vi "Launch Service Mode.vi"(8 "error in (no error)":errorcluster, 11 "Top in":refnum<class "Top.lvclass">) -> (0 "error out":errorcluster, 3 "Top out":refnum<class "Top.lvclass">)   [LabVIEW 2021, in "Top.lvlib" / "Top.lvclass"]
uses:
  Top.lvclass
  Top.lvclass/Top.ctl
  <vilib>/MGI/Panel Manager/Panel Actor/Panel Actor/Panel Actor.lvclass
  <vilib>/MGI/Panel Manager/Panel/Panel.lvlib
  <vilib>/MGI/Panel Manager/Panel/Panel/Window/Window.vi
  <vilib>/MGI/Panel Manager/Panel/Panel/Window/Window.lvclass
  Service/Service.lvclass
  C:/Program Files/National Instruments/LabVIEW 2021/vi.lib/MGI/Panel Manager/Panel/Panel/Panel.lvclass
  C:/Program Files/National Instruments/LabVIEW 2021/vi.lib/MGI/Panel Manager/Panel/Panel/Window/Window.lvclass
  C:/Program Files/National Instruments/LabVIEW 2021/vi.lib/MGI/Panel Manager/Panel Actor/Panel Actor/Panel Actor.lvclass
  C:/Program Files/National Instruments/LabVIEW 2021/vi.lib/ActorFramework/Actor/Actor.lvclass
  C:/git/IV-Curve-PH316/Source/Service/Service.lvclass
  C:/git/IV-Curve-PH316/Source/Top/Top.lvclass
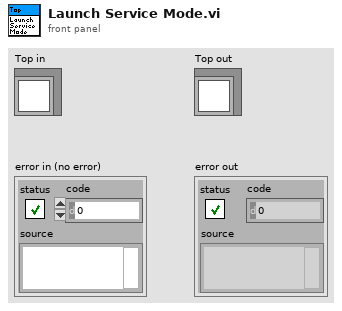
[diagram p1: front panel]
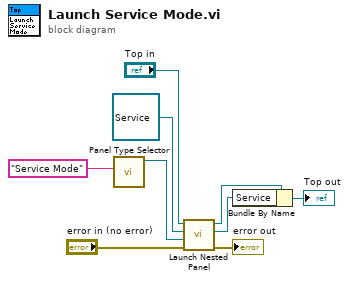
[diagram p0: block diagram]
diagram:
  n1 = call-poly <vilib>:"Panel Type Selector.vi"("Default Title"="Service Mode") -> ("Window out"=w8:refnum<class "Window.lvclass">)  [unwired: 9 in, 1 out]
  n2 = call <vilib>:"Launch Nested Panel.vi"("error in (no error)"="error in (no error)", "Panel"=w8, "Nested Panel Actor"=refnum<class "Service.lvclass"> refnum ("Service.lvlib:Service.lvclass"), "Panel Actor in"="Top in") -> ("error out"=→"error out":errorcluster, "Nested Actor's Enqueuer"=w6:refnum<class "Message Enqueuer.lvclass">, "Panel Actor out"=w9:refnum<class "Top.lvclass">)  [unwired: 4 in, 1 out]
  n3 = Bundle By Name(cluster=w9, "Service"=w6) -> (→"Top out":refnum<class "Top.lvclass">)
